vi "LoggerTest.vi"() -> ()   [LabVIEW 2011]
uses:
  Logger.lvclass
panel:
  in  "Data storage folder":path=path ""
  out "File path out":path
  in  "Array":string[](array[string])
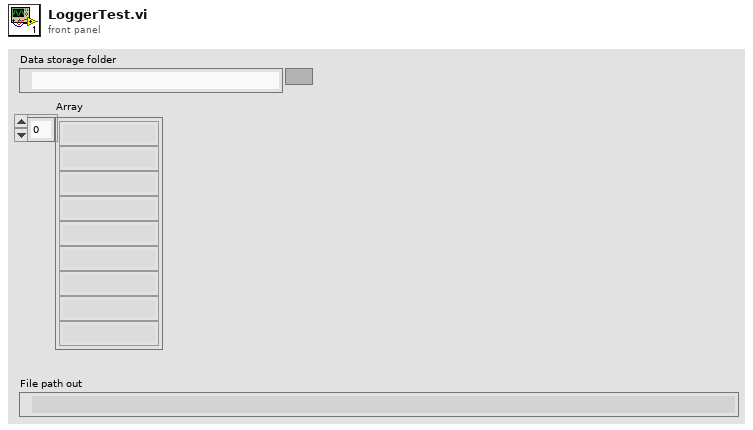
[diagram p1: front panel]
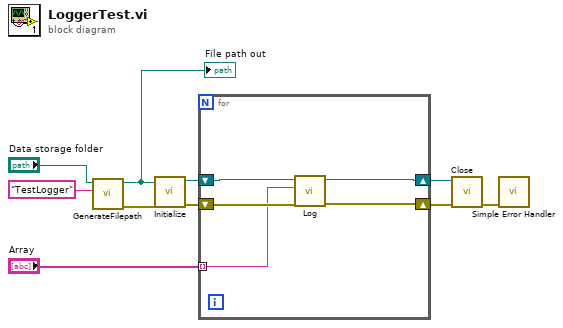
[diagram p0: block diagram]
diagram:
  n1 = call "GenerateFilepath.vi"("Identifier"="TestLogger", "Data storage folder"="Data storage folder") -> ("error out"=w3:errorcluster, "File path out"=w2:path)  [unwired: 8 in]
  "File path out" <- w2
  n2 = call "Initialize.vi"("error in (no error)"=w3, "File path"=w2) -> ("error out"=w8:errorcluster, "Logger out"=w10:refnum<class "Logger.lvclass">)  [unwired: 8 in]
  n3 = for {
    shift-right: [w14] -> w9
    shift-left: w10 -> [w15]
    shift-right: [w12] -> w6
    shift-left: w8 -> [w13]
    tunnel: "Array" -> [w11] mode=indexing
    n4 = call "Log.vi"("error in (no error)"=w13, "Message"=w11, "Logger in"=w15) -> ("error out"=w12:errorcluster, "Logger out"=w14:refnum<class "Logger.lvclass">)  [unwired: 7 in]
  }
  n5 = call "Close.vi"("error in (no error)"=w6, "NetworkStreamWriter in"=w9) -> ("error out"=w5:errorcluster)  [unwired: 9 in]
  n6 = call <vilib>:"Simple Error Handler.vi"("error in (no error)"=w5) -> ()  [unwired: 4 in, 5 out]
